vi "Configure Trigger (Video).vi"(0 "VISA resource name":refnum<visa-resource-name>, 1 "Video Standard (0: NTSC)":i32(ring) items=["NTSC", "PAL"], 2 "Line Number (1)":dbl=1.0, 5 "Trigger Source (0: Channel 1)":i32(ring) items=["Channel 1", "Channel 2", "Channel 3", "Channel 4", "External Input", "Attenuated External Input"], 7 "Polarity (0: Normal)":i32(ring) items=["Normal", "Inverted"], 9 "Sync Condition (0: Field)":i32(ring) items=["Field", "Line", "Odd", "Even", "Line Number"], 11 "error in (no error)":errorcluster) -> (4 "VISA resource out":refnum<visa-resource-name>, 15 "error out":errorcluster)   [LabVIEW 2012, in "Tektronix TDS 200 1000 2000 Series.lvlib"]
doc: "Configures video triggering on the oscilloscope. Video triggering displays NTSC or PAL/SECAM standard composite video waveforms, and is triggered on fields or lines of video signals."
uses:
  <instrlib>/Tektronix TDS 200 1000 2000 Series/Tektronix TDS 200 1000 2000 Series.lvlib
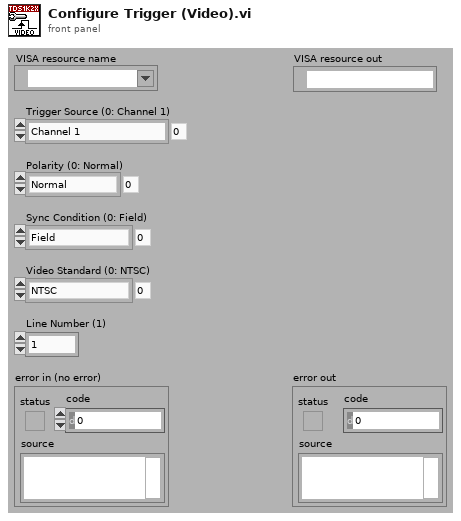
[diagram p1: front panel]
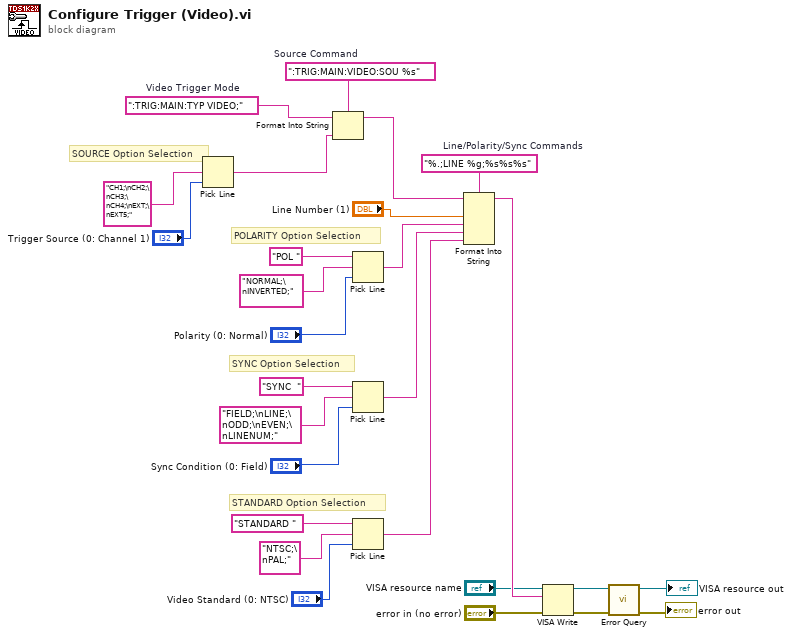
[diagram p0: block diagram]
diagram:
  w25 = "%.;LINE %g;%s%s%s"  # Line/Polarity/Sync Commands
  w27 = ":TRIG:MAIN:TYP VIDEO;"  # Video Trigger Mode
  w26 = ":TRIG:MAIN:VIDEO:SOU %s"  # Source Command
  # "SOURCE Option Selection"
  # "STANDARD Option Selection"
  # "SYNC Option Selection"
  # "POLARITY Option Selection"
  n1 = Pick Line(multi-line string="CH1;\nCH2;\nCH3;\nCH4;\nEXT;\nEXT5;", line index="Trigger Source (0: Channel 1)") -> (output string=w1:string)  [unwired: 1 out]
  n2 = Format Into String(format string=w26, initial string=w27, w1) -> (resulting string=w9:string)  [unwired: 1 in, 1 out]
  n3 = Pick Line(string ("")="POL ", multi-line string="NORMAL;\nINVERTED;", line index="Polarity (0: Normal)") -> (output string=w21:string)
  n4 = Pick Line(string ("")="SYNC  ", multi-line string="FIELD;\nLINE;\nODD;\nEVEN;\nLINENUM;", line index="Sync Condition (0: Field)") -> (output string=w17:string)
  n5 = Pick Line(string ("")="STANDARD ", multi-line string="NTSC;\nPAL;", line index="Video Standard (0: NTSC)") -> (output string=w4:string)
  n6 = Format Into String(format string=w25, initial string=w9, "Line Number (1)", w21, w17, w4) -> (resulting string=w16:string)  [unwired: 1 in, 1 out]
  n7 = VISA Write(VISA resource name="VISA resource name", write buffer=w16, error in (no error)="error in (no error)") -> (VISA resource name out=w23:refnum<visa-resource-name>, error out=w22:errorcluster)  [unwired: 1 out]
  n8 = call <instrlib>:"Error Query.vi"("error in (no error)"=w22, "VISA resource name"=w23) -> ("error out"=→"error out":errorcluster, "VISA resource name out"=→"VISA resource out":refnum<visa-resource-name>)  [unwired: 8 out]
